vi "FP PC main.vi"() -> ()   [LabVIEW 2014]
panel:
  in  "Tab Control":enum32{"Front Page", "Mission Definition"}(tab)
  in  "stop":bool
  in  "Tug letter":string="G"
  out "UDP Time Out?":bool
  out "Blink":bool
  out "error IO":errorcluster
  out "GPS":cluster{"X pos":i32, "Y pos":i32, "Heading":dbl}
  out "Grid Image":T1(plugin-control)
  in  "Pool image\nfile name":string="leds in brightfield cropped.bmp"
  in  "Boat image\nfile name":string="large boat image.png"
  out "Occupancy Grid":u32[][](array[numeric])
  out "Buoy locations":cluster{"regular expression":string, i32, i32}[](array[cluster])
  out "GPS?":bool
  in  "MDF Control":T2(array[cluster])=[{"Type"=enum."Start", "X"=100, "Y"=100, "Speed"=10, "Behaviors"=enum."Open Water Transit"}, {"Type"=enum."Waypoint", "X"=516, "Y"=516, "Speed"=20, "Behaviors"=enum."Open Water Transit"}, {"Type"=enum."Waypoint", "X"=800, "Y"=800, "Speed"=20, "Behaviors"=enum."Open Water Transit"}, {"Type"=enum."End", "X"=0, "Y"=0, "Speed"=0, "Behaviors"=enum."Open Water Transit"}]
  # "This page is used to plan the mission.  The MDF, Mission Definition File, control below is used for that purpose.\n\n*  Each mission must begin with a record of type \"Start\" and end with a record of type \"End\"\n*  For the \"Start\" and \"End\" records the remaining entries have no impact.\n*  For the \"Waypoint\" records you must set a position for the waypoint, a speed, and a behavior.\n*  Any number of records may be used.\n*  The simulation will place a \"yellow\" marker at the local of each waypoint include.\n*  If you declare unused records type \"End\" they will not be include in the simulation"
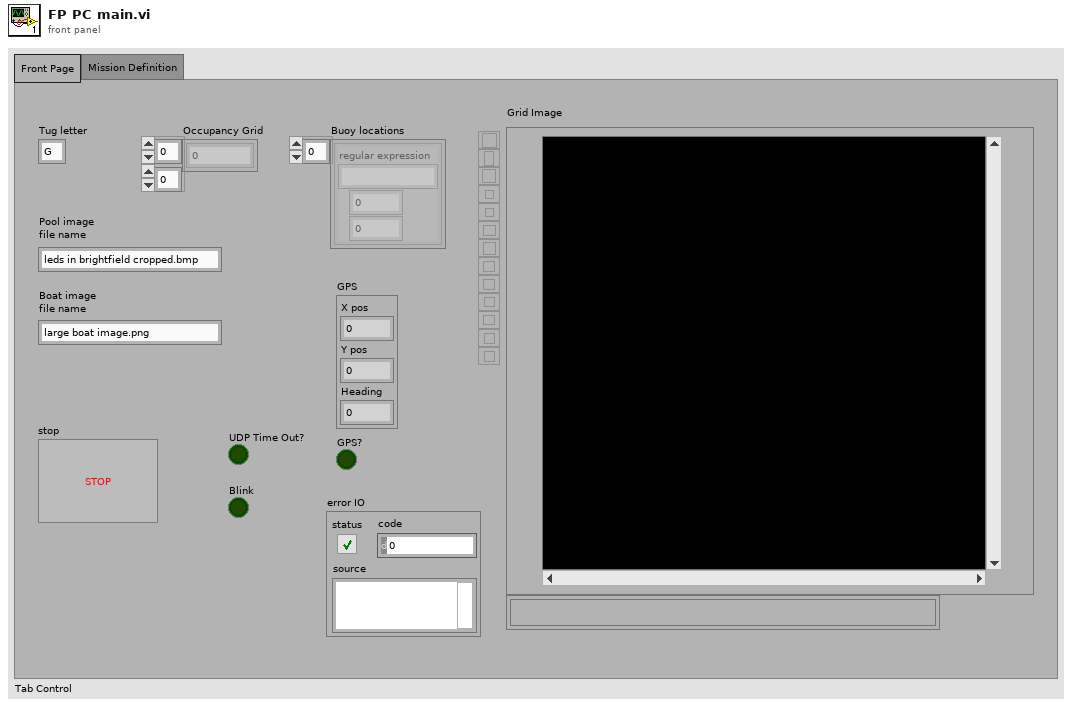
[diagram p1: front panel]
types:
  T1 = typedef "IMAQ Image.ctl" = refnum<image>
  T2 = cluster{"Type":enum16{"Start", "Waypoint", "End"}, "X":i32, "Y":i32, "Speed":i32, "Behaviors":enum16{"Open Water Transit", "P-Wall Follow", "S-Wall Follow", "Dock"}}[]
  T3 = typedef "Image Type" = u32
  T4 = cluster{"regular expression":string, i32, i32, i32}
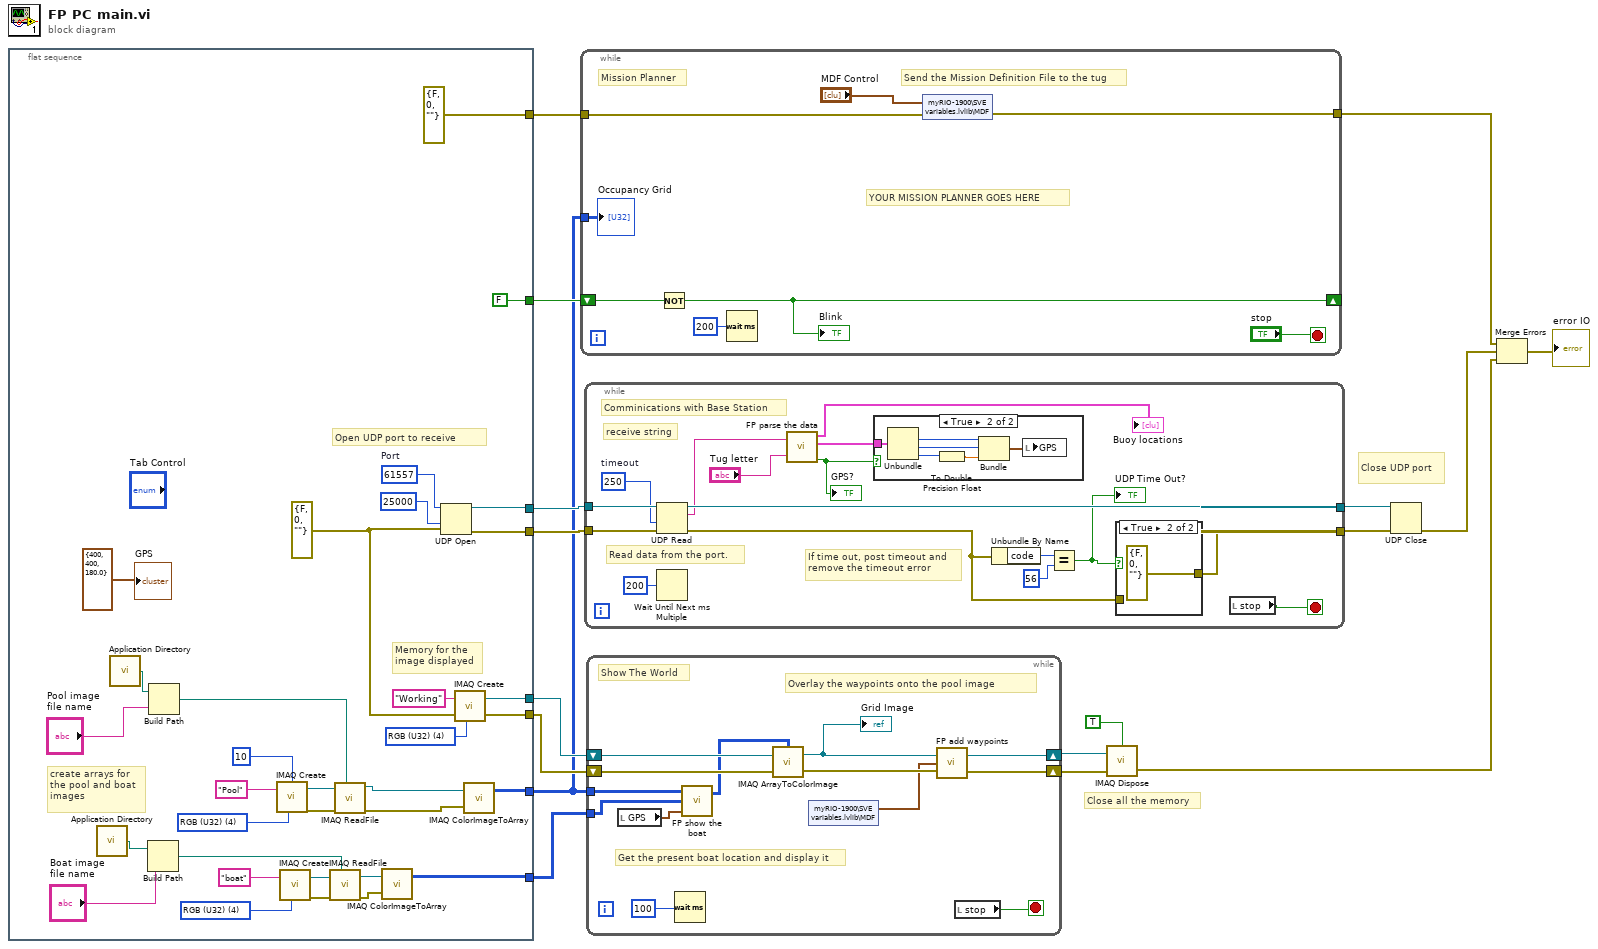
[diagram p0: block diagram]
diagram:
  # "Close all the memory"
  # "Close UDP port"
  n1 = flat-sequence {
    tunnel: [errorcluster {"status"=FALSE, "code"=0, "source"=""} ("error in (no error)")] -> w17
    tunnel: [w47] -> w14
    tunnel: [w46] -> w13
    tunnel: [FALSE] -> w9
    tunnel: [w23] -> w5
    tunnel: [w22] -> w1
    tunnel: [w21] -> w4
    tunnel: [w20] -> w3
    frame #0 {
      w35 = T3 4 items=["Grayscale (U8)", "Grayscale (I16)", "Grayscale (SGL)", "Complex (CSG)", "RGB (U32)", "HSL (U32)", "RGB (U64)", "Grayscale (U16)"] ("Image Type")
      w31 = T3 4 items=["Grayscale (U8)", "Grayscale (I16)", "Grayscale (SGL)", "Complex (CSG)", "RGB (U32)", "HSL (U32)", "RGB (U64)", "Grayscale (U16)"] ("Image Type")
      w27 = T3 4 items=["Grayscale (U8)", "Grayscale (I16)", "Grayscale (SGL)", "Complex (CSG)", "RGB (U32)", "HSL (U32)", "RGB (U64)", "Grayscale (U16)"] ("Image Type")
      w19 = errorcluster {"status"=FALSE, "code"=0, "source"=""} ("error in (no error)")
      w48 = u16 61557  # Port
      # "Memory for the\nimage displayed"
      # "create arrays for\nthe pool and boat\nimages"
      # "Open UDP port to receive"
      n2 = call <vilib>:"Application Directory.vi"() -> ("Application Directory"=w42:path)
      n3 = call <vilib>:"Application Directory.vi"() -> ("Application Directory"=w41:path)
      n4 = Build Path(base path=w42, name or relative path="Boat image\nfile name") -> (appended path=w44:path)
      n5 = Build Path(base path=w41, name or relative path="Pool image\nfile name") -> (appended path=w39:path)
      n6 = call "IMAQ Create"("Border Size"=10, "Image Name"="Pool", "Image Type"=w27) -> ("New Image"=w25:T1, "error out"=w26:errorcluster)  [unwired: 2 in]
      n7 = call "IMAQ Create"("Image Name"="boat", "Image Type"=w31) -> ("New Image"=w29:T1, "error out"=w30:errorcluster)  [unwired: 3 in]
      n8 = call "IMAQ ReadFile"("File Path"=w44, "error in (no error)"=w30, "Image"=w29) -> ("error out"=w33:errorcluster, "Image Out"=w34:T1)  [unwired: 4 in, 3 out]
      n9 = call "IMAQ ReadFile"("File Path"=w39, "error in (no error)"=w26, "Image"=w25) -> ("error out"=w38:errorcluster, "Image Out"=w37:T1)  [unwired: 4 in, 3 out]
      n10 = call "IMAQ ColorImageToArray"("Image"=w34, "error in (no error)"=w33) -> ("Image Pixels (U32)"=w23:u32[][])  [unwired: 2 in, 2 out]
      n11 = UDP Open(8:w19, 9:25000 ("timeout ms (25000)"), 11:w48) -> (port=w46:refnum<k16>, 0:w47:errorcluster)  [unwired: 2 in, 1 out]
      n12 = call "IMAQ Create"("Image Name"="Working", "Image Type"=w35, "error in (no error)"=w19) -> ("New Image"=w21:T1, "error out"=w20:errorcluster)  [unwired: 2 in]
      n13 = call "IMAQ ColorImageToArray"("Image"=w37, "error in (no error)"=w38) -> ("Image Pixels (U32)"=w22:u32[][])  [unwired: 2 in, 2 out]
      "GPS" <- cluster{i32, i32, dbl} {400, 400, 180.0} ("output cluster")
    }
  }
  n14 = while {
    tunnel: w17 -> [w54]
    tunnel: [w56] -> w11
    shift-right: [w52] -> _
    shift-left: w9 -> [w53]
    tunnel: w1 -> [w51]
    stop <- "stop" stop-if-true
    # "Send the Mission Definition File to the tug"
    # "YOUR MISSION PLANNER GOES HERE"
    # "Mission Planner"
    n15 = Not(x=w53) -> (.not. x?=w52:bool)
    "Blink" <- w52
    n16 = Wait (ms)(milliseconds to wait=u32 200) -> ()  [unwired: 1 out]
    n17 = shared-variable "myRIO-1900\\SVE variables.lvlib\\MDF"("MDF Control", error in=w54) -> (error out=w56:errorcluster)
    "Occupancy Grid" <- w51
  }
  n18 = while {
    tunnel: w14 -> [w74]
    tunnel: w13 -> [w73]
    tunnel: [w72] -> w16
    tunnel: [w67] -> w15
    stop <- w64 stop-if-true
    w66 = 250  # timeout
    # "Comminications with Base Station"
    # "receive string"
    # "If time out, post timeout and\nremove the timeout error"
    # "Read data from the port."
    n19 = UDP Read(connection ID=w73, timeout ms (25000)=w66, 8:w74) -> (data out=w61:string, error out=w68:errorcluster, 3:w72:refnum<k16>)  [unwired: 1 in, 2 out]
    n20 = Wait Until Next ms Multiple(millisecond multiple=u32 200) -> ()  [unwired: 1 out]
    n21 = call "FP parse the data.vi"("Nav String"=w61, "Tug"="Tug letter") -> ("Buoy locations"=→"Buoy locations":cluster{"regular expression":string, i32, i32}[], "Tug Location"=w62:T4, "Valid?"=w59:bool)  [unwired: 1 out]
    "GPS?" <- w59
    n22 = case shown="True" w59 {
      tunnel: w62 -> [_ w80]
      frame False {
      }
      frame True {
        n23 = Unbundle(w80) -> (w79:i32, w78:i32, w76:i32)  [unwired: 1 out]
        n24 = To Double Precision Float(number=w76) -> (double precision float=w77:dbl)
        n25 = Bundle(w79, w78, w77) -> (w75:cluster{i32, i32, dbl})  [unwired: 1 in]
        n26 = local write "GPS"(w75) -> ()
      }
    }
    n27 = Unbundle By Name(w68) -> ("code"=w71:i32)
    n28 = Equal?(x=w71, y=56) -> (x = y?=w69:bool)
    "UDP Time Out?" <- w69
    n29 = case shown="True" w69 {
      tunnel: [w81 errorcluster {"status"=FALSE, "code"=0, "source"=""} ("error out")] -> w67
      tunnel: w68 -> [w81 _]
      frame False {
      }
      frame True {
      }
    }
    n30 = local read "stop"() -> (w64:bool)
  }
  n31 = while {
    tunnel: w5 -> [w87]
    tunnel: w1 -> [w88]
    shift-right: [w89] -> w7
    shift-left: w3 -> [w95]
    shift-right: [w90] -> w6
    shift-left: w4 -> [w94]
    stop <- w93 stop-if-true
    # "Overlay the waypoints onto the pool image"
    # "Show The World"
    # "Get the present boat location and display it"
    n32 = local read "GPS"() -> (w85:cluster{"X pos":i32, "Y pos":i32, "Heading":dbl})
    n33 = Wait (ms)(milliseconds to wait=u32 100) -> ()  [unwired: 1 out]
    n34 = call "FP show the boat.vi"("GPS"=w85, "Boat array"=w87, "Pool array"=w88) -> ("Pool out"=w84:u32[][])  [unwired: 1 in]
    n35 = call "IMAQ ArrayToColorImage"("Image Pixels (U32)"=w84, "Image"=w94, "error in (no error)"=w95) -> ("Image Out"=w91:T1, "error out"=w92:errorcluster)  [unwired: 2 in]
    "Grid Image" <- w91
    n36 = shared-variable "myRIO-1900\\SVE variables.lvlib\\MDF"() -> (w83:T2)  [unwired: 1 in, 1 out]
    n37 = call "FP add waypoints.vi"("error in"=w92, "MDF Control"=w83, "Image In"=w91) -> ("error out"=w89:errorcluster, "Image Out"=w90:T1)
    n38 = local read "stop"() -> (w93:bool)
  }
  n39 = call "IMAQ Dispose"("All Images? (No)"=TRUE, "Image"=w6, "error in (no error)"=w7) -> ("error out"=w2:errorcluster)  [unwired: 3 in]
  n40 = UDP Close(connection ID=w16, 8:w15) -> (error out=w12:errorcluster)  [unwired: 1 out]
  n41 = Merge Errors(w11, w12, w2) -> (→"error IO":errorcluster)
